vi "ChangeDriveTrainDeadband.vi"(10 "Eliminate Deadband":bool, 11 "Drivetrain in":T1) -> (3 "Drivetrain out":T1)   [LabVIEW 2016]
uses:
  <vilib>/Rock Robotics/WPI/RobotDrive/WPI_RobotDriveDevRef.ctl
  <vilib>/Rock Robotics/WPI/MotorControl/WPI_MotorControlDeviceRef.ctl
  <vilib>/Rock Robotics/WPI/MotorControl/WPI_MotorControlType.ctl
  <vilib>/Rock Robotics/SystemInterfaces/DIO/FPGA_DIOPWMChannel.ctl
  <vilib>/Rock Robotics/WPI/PWM/WPI_PWMDeadband.ctl
  <vilib>/Rock Robotics/WPI/PWM/WPI_PWMDeadband_ms.ctl
  Constants/Private/Private Global.vi
  Constants/Constants.lvlib
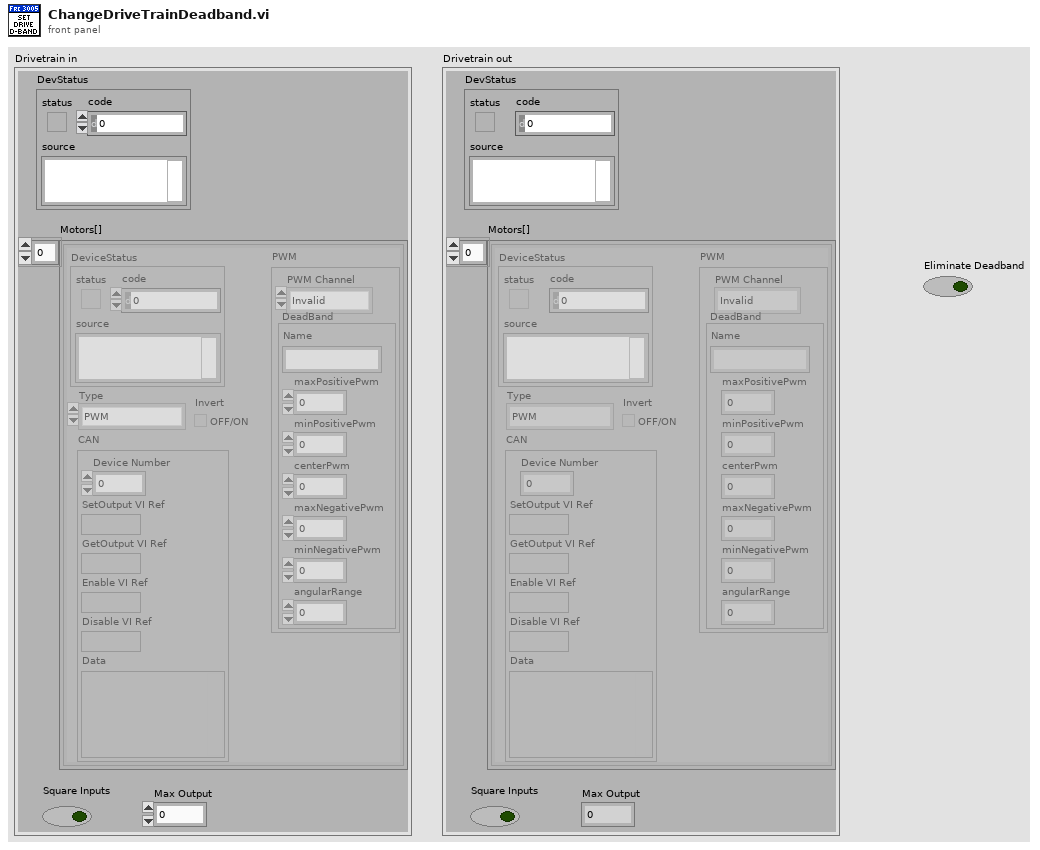
[diagram p1: front panel]
types:
  T1 = typedef "WPI_RobotDriveDevRef.ctl" = cluster{"DevStatus":errorcluster, "Motors[]":T2[], "Square Inputs":bool, "Max Output":dbl}
  T2 = typedef "WPI_MotorControlDeviceRef.ctl" = cluster{"DeviceStatus":errorcluster, "Type":T3, "PWM":cluster{"PWM Channel":T4, "DeadBand":T5}, "CAN":cluster{"Device Number":u8, "SetOutput VI Ref":variant, "GetOutput VI Ref":variant, "Enable VI Ref":variant, "Disable VI Ref":variant, "Data":variant}, "Invert":bool}
  T3 = typedef "WPI_MotorControlType.ctl" = enum16{"PWM", "CAN"}
  T4 = typedef "FPGA_DIOPWMChannel.ctl" = enum8{"PWM 0", "PWM 1", "PWM 2", "PWM 3", "PWM 4", "PWM 5", "PWM 6", "PWM 7", "PWM 8", "PWM 9", "PWM MXP 0", "PWM MXP 1", "PWM MXP 2", "PWM MXP 3", "PWM MXP 4", "PWM MXP 5", "PWM MXP 6", "PWM MXP 7", "PWM MXP 8", "PWM MXP 9", "Invalid"}
  T5 = typedef "WPI_PWMDeadband.ctl" = cluster{"Name":string, "maxPositivePwm":i32, "minPositivePwm":i32, "centerPwm":i32, "maxNegativePwm":i32, "minNegativePwm":i32, "angularRange":u16}
  T6 = typedef "Constants.lvlib/Constants.ctl" = cluster{"Port Layout":cluster{"RightMotorInverted":bool, "LeftMotorInverted":bool, "Left Motors":T4, "Right Motors":T4, "Auton List":string[], "XBOX Port":T7, "Encoder L A":T8, "Encoder L B":T8, "Encoder R A":T8, "Encoder R B":T8, "L Encoder Inverse":bool, "R Encoder Inverse":bool, "Drive Distance per Count":dbl, "Gyro Bus":T9, "Fuel Roller 1":T4, "Front Roller":T4, "Gear Flipper":T4, "Climber 1":T4, "Fuel Roller Invert":bool, "Front Roller Invert":bool, "Gear Flipper Invert":bool, "Climber Invert":bool, "PCM":u8, "Fuel Roller 2":T4, "Gear Sensor":T10, "Gear Release Fwd":T11, "Gear Release Rvrs":T11, "Fuel Arm Fwd":T11, "Fuel Arm Rvrs":T11, "Shifter Fwrd":T11, "Shifter Rvrs":T11, "Climber 2":T4, "PDP":u8, "Shooter Front Channel":u8, "Shooter Rear Channel":u8, "Shooter Feed Channel":u8, "Camera Servo":T4, "Gear Servo":T4, "Gear Puncher Fwrd":T11, "Gear Puncher Rvrs":T11, "Shooter Inverse":bool, "Ring Light Switch":T8}, "Drive Constants":cluster{"Wheelbase In.":dbl, "Max Velocity (In/sec)":dbl, "Max Accel (In/sec^2)":dbl, "Max Jerk (In/sec^3)":dbl, "Path dt":dbl, "Path Sample Count":i32, "Deadband":dbl}, "Arm System":cluster{"Front Roller Gear Speed":dbl, "Front Roller Fuel Speed":dbl, "Gear Flipper Speed":dbl, "Fuel Roller Speed":dbl, "Gear Release Wait (ms)":i32, "Gear Sensor Threshold":dbl, "Flappy Open Angle":i32, "Flappy Close Angle":i32, "Ramp Rate (EGU/min)":dbl}, "Shooter":cluster{"Shooter Wheels":cluster{"P":dbl, "I":dbl, "D":dbl, "F":dbl, "IZone":dbl}, "Feeder":cluster{"P":dbl, "I":dbl, "D":dbl, "F":dbl, "IZone":dbl}, "Front Shooter RPM":dbl, "Rear Shooter RPM":dbl, "Agitator Speed":dbl, "Feeder Speed":dbl, "Shooter CPR":u32, "Feeder CPR":u32}, "Vision":cluster{"High Goal Height (in.)":dbl, "Low Goal Height (in.)":dbl, "Camera Height High (in.)":dbl, "Camera Height Low (in.)":dbl, "Servo Pitch Gear (deg)":dbl, "Camera Yaw (deg)":dbl, "Servo Gear":i32, "Servo Boiler":i32, "Servo Pitch Boiler (deg)":dbl}}
  T7 = typedef "WPI_JoystickDeviceEnum.ctl" = enum16{"USB 0", "USB 1", "USB 2", "USB 3", "USB 4", "USB 5"}
  T8 = typedef "FPGA_DIOChannel.ctl" = enum8{"DIO 0", "DIO 1", "DIO 2", "DIO 3", "DIO 4", "DIO 5", "DIO 6", "DIO 7", "DIO 8", "DIO 9", "DIO MXP 0", "DIO MXP 1", "DIO MXP 2", "DIO MXP 3", "DIO MXP 4", "DIO MXP 5", "DIO MXP 6", "DIO MXP 7", "DIO MXP 8", "DIO MXP 9", "DIO MXP 10", "DIO MXP 11", "DIO MXP 12", "DIO MXP 13", "DIO MXP 14", "DIO MXP 15", "SPI Port CS1", "SPI Port CS2", "SPI Port CS3", "SPI Port MISO", "SPI Port MOSI", "Invalid"}
  T9 = typedef "spi_bus.ctl" = enum16{"SPI On-Board, CS0", "SPI On-Board, CS1", "SPI On-Board, CS2", "SPI On-Board, CS3", "SPI MXP", "Invalid"}
  T10 = typedef "FPGA_AIChannel.ctl" = enum8{"AI 0", "AI 1", "AI 2", "AI 3", "AI MXP 0", "AI MXP 1", "AI MXP 2", "AI MXP 3", "Invalid"}
  T11 = typedef "WPI_SolenoidChannel.ctl" = enum8{"Solenoid 0", "Solenoid 1", "Solenoid 2", "Solenoid 3", "Solenoid 4", "Solenoid 5", "Solenoid 6", "Solenoid 7", "Invalid"}
  T12 = typedef "WPI_PWMDeadband_ms.ctl" = cluster{"Name":string, "maxPositivePwm":dbl, "minPositivePwm":dbl, "centerPwm":dbl, "maxNegativePwm":dbl, "minNegativePwm":dbl}
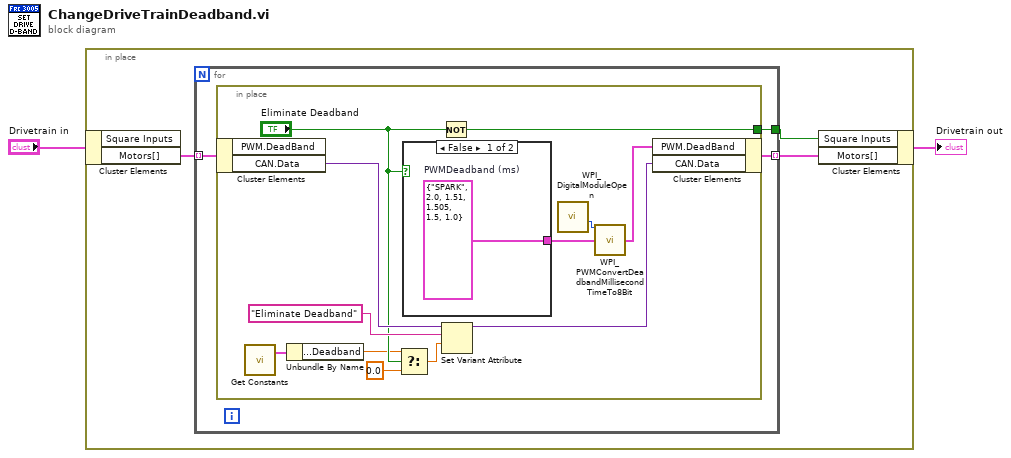
[diagram p0: block diagram]
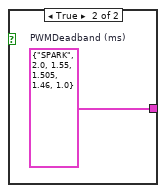
[diagram p2: hidden frame]
diagram:
  n1 = in-place {
    n2 = in-place-cluster #1("Drivetrain in") -> ("Motors[]"=w5:T2[])  [unwired: 1 out]
    n3 = for {
      tunnel: w5 -> [w8] mode=indexing
      tunnel: [w7] -> w4 mode=indexing
      tunnel: [w6] -> w3
      n4 = in-place {
        in-place-border: [w17] -> w6
        n5 = in-place-cluster #2(w8) -> ("CAN.Data"=w16:variant)  [unwired: 1 out]
        n6 = call "Get Constants.vi"() -> ("Constants"=w10:T6)  [unwired: 3 in]
        n7 = Unbundle By Name(w10) -> ("Drive Constants.Deadband"=w9:dbl)
        n8 = Select(t=w9, s="Eliminate Deadband", f=0.0) -> (s? t:f=w12:dbl)
        n9 = case shown="False" "Eliminate Deadband" {
          tunnel: [w21 w22] -> w20
          frame False {
            w21 = T12 {"Name"="SPARK", "maxPositivePwm"=2.0, "minPositivePwm"=1.51, "centerPwm"=1.505, "maxNegativePwm"=1.5, "minNegativePwm"=1.0}  # PWMDeadband (ms)
          }
          frame True {
            w22 = T12 {"Name"="SPARK", "maxPositivePwm"=2.0, "minPositivePwm"=1.55, "centerPwm"=1.505, "maxNegativePwm"=1.46, "minNegativePwm"=1.0}  # PWMDeadband (ms)
          }
        }
        n10 = Not(x="Eliminate Deadband") -> (.not. x?=w17:bool)
        n11 = Set Variant Attribute(Variant=w16, name="Eliminate Deadband", value=w12) -> (Variant out=w14:variant)  [unwired: 1 in, 2 out]
        n12 = call <vilib>:"WPI_DigitalModuleOpen.vi"() -> ("LoopTiming"=w18:u16)  [unwired: 2 in, 9 out]
        n13 = call <vilib>:"WPI_PWMConvertDeadbandMillisecondTimeTo8Bit.vi"("DIO Loop Timing (ticks)"=w18, "PWMDeadband (ms)"=w20) -> ("PWMDeadband Coefficient"=w19:T5)  [unwired: 13 in]
        n14 = in-place-cluster #2("PWM.DeadBand"=w19, "CAN.Data"=w14) -> (w7:T2)
      }
    }
    n15 = in-place-cluster #1("Square Inputs"=w3, "Motors[]"=w4) -> (→"Drivetrain out":T1)
  }
